vi "Refresh Mappings.vi"(8 "error in (no error)":errorcluster, 10 "Destination to Highlight":string, 11 "Loop Data":T1) -> (0 "error out":errorcluster)   [LabVIEW 2016, in "System Mapping Tool.lvlib"]
uses:
  System Mapping Tool.lvlib
  TypeDefs/Loop Data.ctl
  TypeDefs/UI Refs.ctl
  NationalInstruments.VeriStand.SystemDefinitionAPI
  NationalInstruments.VeriStand.SystemStorageUI
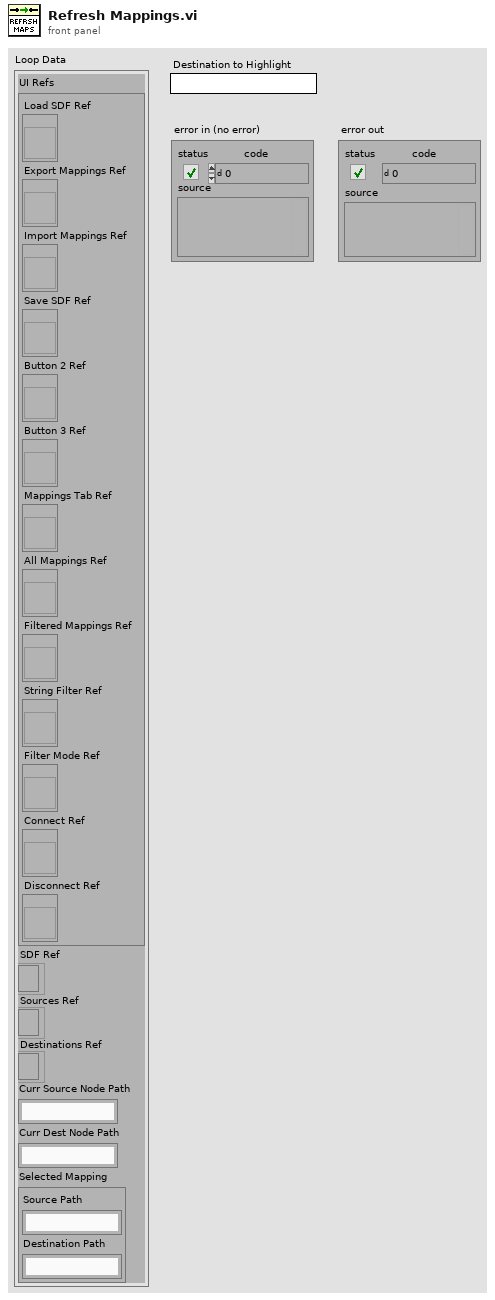
[diagram p1: front panel]
types:
  T1 = typedef "System Mapping Tool.lvlib/Loop Data.ctl" = cluster{"UI Refs":T2, "SDF Ref":refnum<k24>, "Sources Ref":refnum<k24>, "Destinations Ref":refnum<k24>, "Curr Source Node Path":string, "Curr Dest Node Path":string, "Selected Mapping":cluster{"Source Path":string, "Destination Path":string}}
  T2 = typedef "System Mapping Tool.lvlib/UI Refs.ctl" = cluster{"Load SDF Ref":refnum<vi>, "Export Mappings Ref":refnum<vi>, "Import Mappings Ref":refnum<vi>, "Save SDF Ref":refnum<vi>, "Button 2 Ref":refnum<vi>, "Button 3 Ref":refnum<vi>, "Mappings Tab Ref":refnum<vi>, "All Mappings Ref":refnum<vi>, "Filtered Mappings Ref":refnum<vi>, "String Filter Ref":refnum<vi>, "Filter Mode Ref":refnum<vi>, "Connect Ref":refnum<vi>, "Disconnect Ref":refnum<vi>}
  T3 = enum32{"All System Mappings", "Filtered Mappings by Node"}
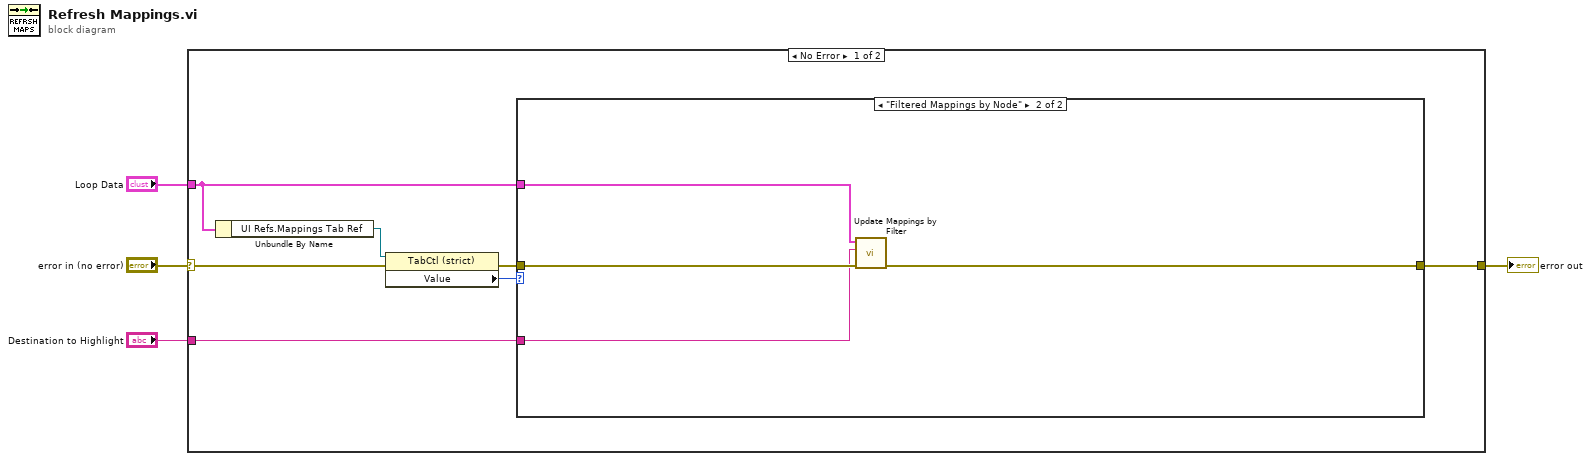
[diagram p0: block diagram]
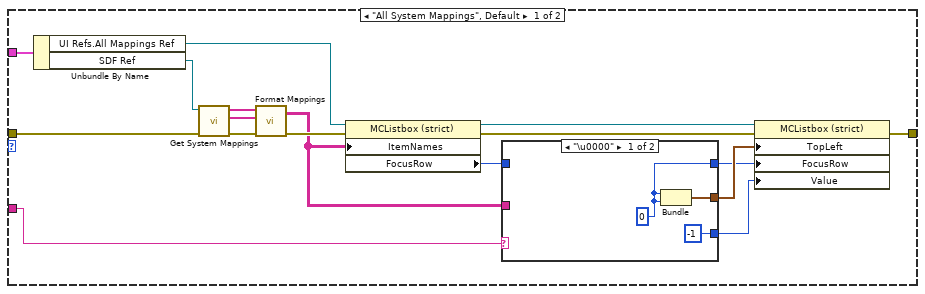
[diagram p2: hidden frame]
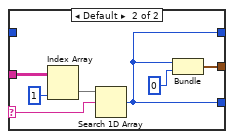
[diagram p3: hidden frame]
diagram:
  n1 = case shown="No Error" "error in (no error)" {
    selector: "error in (no error)" -> [w11 w42]
    tunnel: [w6 w42] -> w3
    tunnel: "Loop Data" -> [w7 _]
    tunnel: "Destination to Highlight" -> [w5 _]
    frame No Error {
      n2 = Unbundle By Name(w7) -> ("UI Refs.Mappings Tab Ref"=w10:refnum<vi>)
      n3 = property class="TabCtl (strict)"(reference=w10, error in=w11) -> (error out=w8:errorcluster, "Value"=w9:T3)  [unwired: 1 out]
      n4 = case shown="\"Filtered Mappings by Node\"" w9 {
        tunnel: w8 -> [w22 w41]
        tunnel: w7 -> [w27 w40]
        tunnel: [w19 w39] -> w6
        tunnel: w5 -> [w12 w38]
        frame "All System Mappings", Default {
          n5 = Unbundle By Name(w27) -> ("UI Refs.All Mappings Ref"=w26:refnum<vi>, "SDF Ref"=w21:refnum<k24>)
          n6 = call "Get System Mappings.vi"("error in (no error)"=w22, "SDF Ref"=w21) -> ("error out"=w23:errorcluster, "Destinations"=w24:string[], "Sources"=w20:string[])  [unwired: 7 in]
          n7 = call "Format Mappings.vi"("Destinations"=w24, "Sources"=w20) -> ("Mappings"=w16:string[][])  [unwired: 3 in]
          n8 = property class="MCListbox (strict)"(reference=w26, error in=w23, "ItemNames"=w16) -> (reference out=w18:refnum<vi>, error out=w25:errorcluster, "FocusRow"=w15:i32)
          n9 = case shown="\"\"" w12 {
            selector: w12 -> [_ w33]
            tunnel: [w30 w32] -> w17
            tunnel: w16 -> [_ w36]
            tunnel: w15 -> [_ _]
            tunnel: [w28 w31] -> w14
            tunnel: [-1 ("index of element") w31] -> w13
            frame "\u0000" {
              w28 = 0
              n10 = Bundle(w28, w28) -> (w30:cluster{i32, i32})  [unwired: 1 in]
            }
            frame Default {
              n11 = Index Array(array=w36, index (col)=1 ("disabled index (col)")) -> (element=w35:string[])  [unwired: 1 in]
              n12 = Search 1D Array(1D array=w35, element=w33) -> (index of element=w31:i32)  [unwired: 1 in]
              n13 = Bundle("index of element"=w31, 0) -> (w32:cluster{"index of element":i32, i32})  [unwired: 1 in]
            }
          }
          n14 = property class="MCListbox (strict)"(reference=w18, error in=w25, "TopLeft"=w17, "FocusRow"=w14, "Value"=w13) -> (error out=w19:errorcluster)  [unwired: 1 out]
        }
        frame "Filtered Mappings by Node" {
          n15 = call "Update Mappings by Filter.vi"("error in (no error)"=w41, "Destination to Highlight"=w38, "Loop Data in"=w40) -> ("error out"=w39:errorcluster)  [unwired: 8 in]
        }
      }
    }
    frame Error {
    }
  }
  "error out" <- w3
